vi "handleSettings.vi"(8 "error in (no error)":errorcluster, 10 "Path":path, 11 "CameraController in":refnum<class "CameraController.lvclass">) -> (0 "error out":errorcluster, 3 "CameraController out":refnum<class "CameraController.lvclass">)   [LabVIEW 2009, in "Hardware.lvlib" / "Channels.lvlib" / "CameraController.lvclass"]
doc: "Override this method in a subclass to load specific settings for the camera being used."
uses:
  CameraController.lvclass
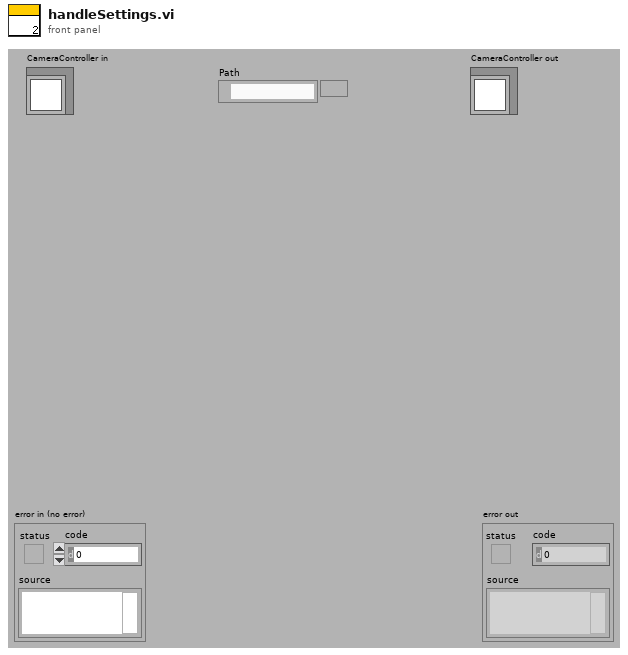
[diagram p1: front panel]
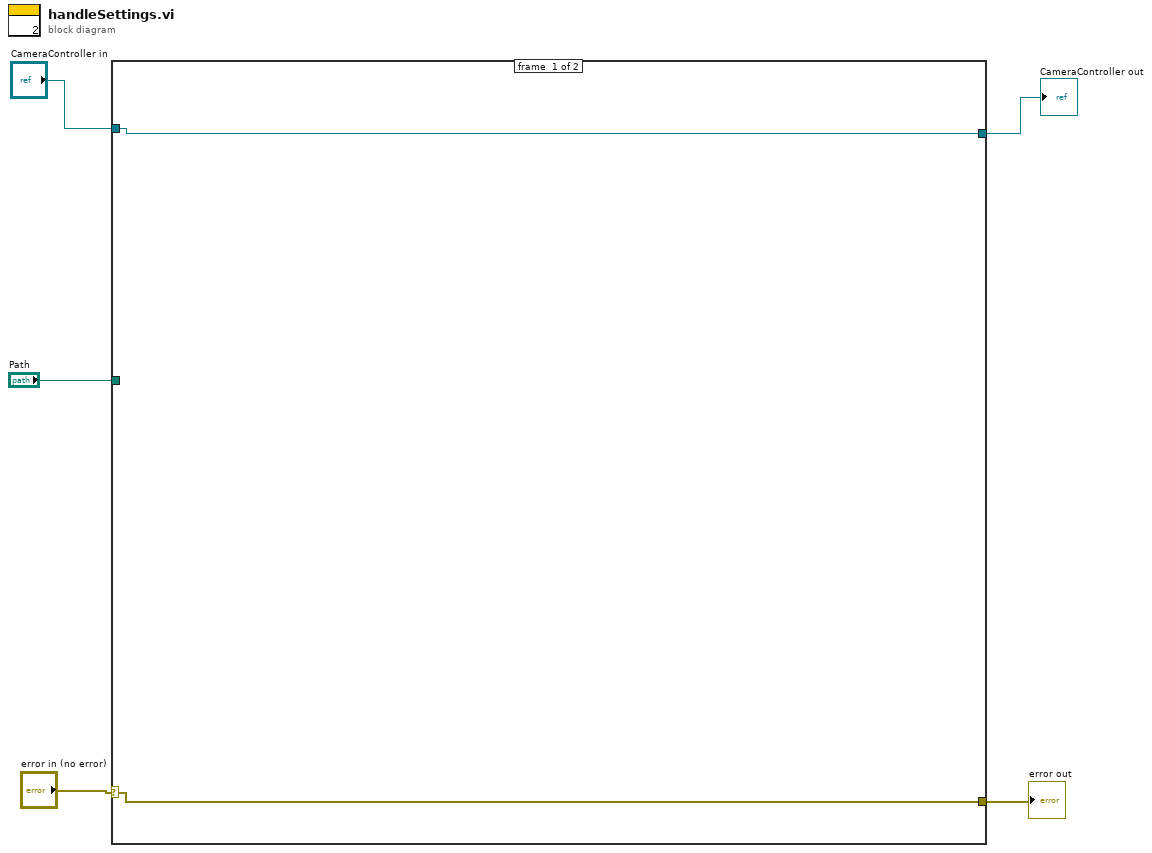
[diagram p0: block diagram]
diagram:
  n1 = case shown="No Error" "error in (no error)" {
    selector: "error in (no error)" -> [w7 w9]
    tunnel: [w7 w9] -> w4
    tunnel: "CameraController in" -> [w6 w8]
    tunnel: [w6 w8] -> w2
    tunnel: "Path" -> [_ _]
    frame #0 {
    }
    frame #1 {
    }
  }
  "error out" <- w4
  "CameraController out" <- w2
